vi "Load App.vi"(8 "error in (no error)":errorcluster) -> (0 "error out":errorcluster)   [LabVIEW 2016, in "User Interface.lvlib" / "User Interface.lvclass"]
uses:
  User Interface.lvclass
  C:/Program Files (x86)/National Instruments/LabVIEW 2016/vi.lib/ActorFramework/Actor/Actor.lvclass
  <vilib>/ActorFramework/Actor/Actor.lvclass
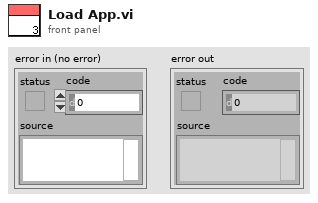
[diagram p1: front panel]
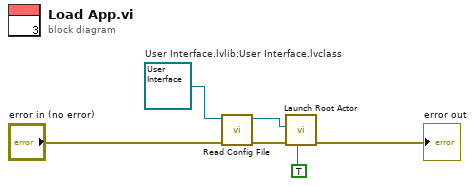
[diagram p0: block diagram]
diagram:
  w3 = refnum<class "User Interface.lvclass"> refnum  # User Interface.lvlib:User Interface.lvclass
  n1 = call-dynamic "Read Config File.vi"("error in (no error)"="error in (no error)", "Trace Grabber Application in"=w3) -> ("Trace Grabber Application out"=w2:refnum<class "User Interface.lvclass">)  [unwired: 8 in, 1 out]
  n2 = call <vilib>:"Launch Root Actor.vi"("Open Actor Core front panel? (F)"=TRUE, "error in (no error)"="error in (no error)", "Actor"=w2) -> ("error out"=→"error out":errorcluster)  [unwired: 7 in, 1 out]
